vi "Database Query Search With Return Value.vi"(8 "error in (no error)":errorcluster, 10 "SQL query":string, 11 "object in":refnum<class "Database.lvclass">) -> (0 "error out":errorcluster, 1 "Not Empty":bool, 2 "recordset data":variant[][](array[variant]), 3 "object out":refnum<class "Database.lvclass">)   [LabVIEW 2015, in "Database.lvclass"]
uses:
  Database.lvclass
  <vilib>/addons/database/Auxilliary.llb/DB Tools Cursor Type.ctl
  Database.lvclass/Database.ctl
  <vilib>/addons/database/Connection.llb/DB Tools Open Connec (String).vi
  <vilib>/addons/database/Connection.llb/Conn Execute.vi
  <vilib>/addons/database/Recordset.llb/Rec Get Recordset Properties (R).vi
  <vilib>/addons/database/Recordset.llb/Rec Fetch Recordset Data (R).vi
  <vilib>/addons/database/Recordset.llb/Rec Destroy - Connection.vi
  <vilib>/addons/database/NI_Database_API.lvlib
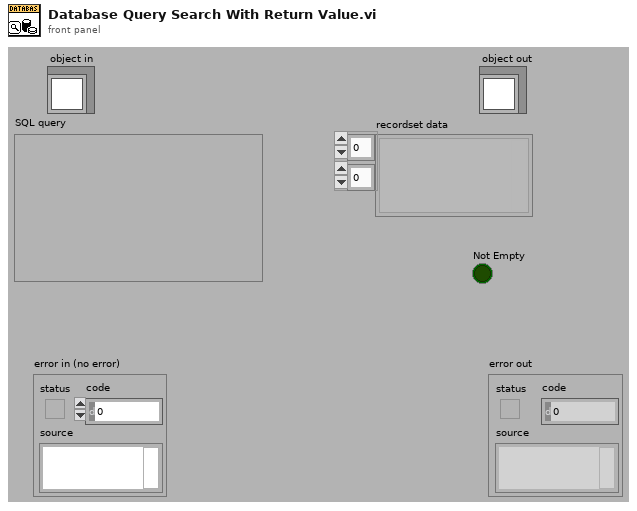
[diagram p1: front panel]
types:
  T1 = typedef "NI_Database_API.lvlib/DB Tools Cursor Type.ctl" = enum16{"forward-only", "keyset", "dynamic", "static"}
  T2 = typedef "NI_Database_API.lvlib/Conn ObjectReference.ctl" = refnum<k1>
  T3 = typedef "NI_Database_API.lvlib/Rec ObjectReference.ctl" = refnum<k1>
  T4 = typedef "NI_Database_API.lvlib/Rec Properties.ctl" = cluster{"column count":i32, "record index":i32, "record count":i32, "bof?":bool, "eof?":bool, "cursor type":T1, "cache size":i32, "state":enum16{"closed", "open"}}
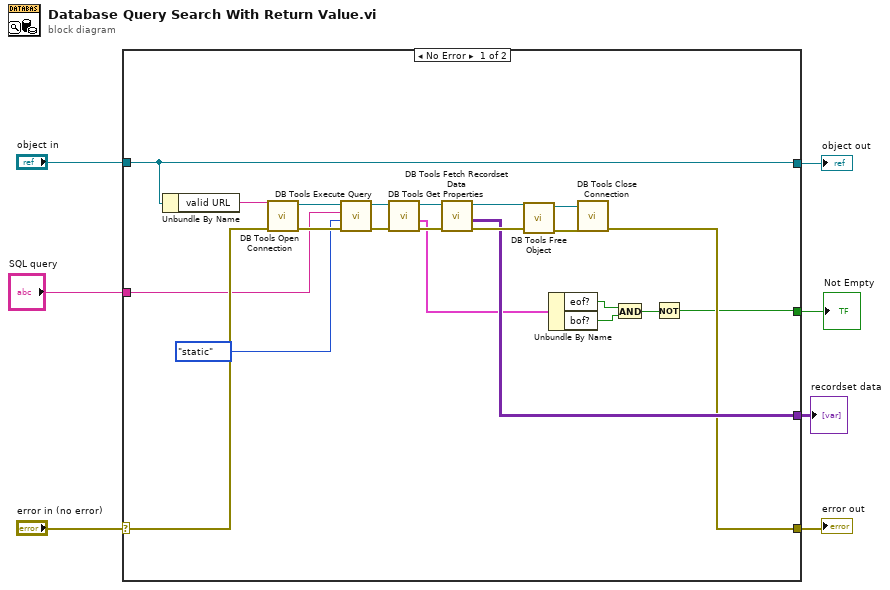
[diagram p0: block diagram]
diagram:
  n1 = case shown="No Error" "error in (no error)" {
    selector: "error in (no error)" -> [w27 w31]
    tunnel: [w17 w31] -> w6
    tunnel: [w29 w30] -> w4
    tunnel: "object in" -> [w29 w30]
    tunnel: "SQL query" -> [w23 _]
    tunnel: [w18 _] -> w2
    tunnel: [w8 _] -> w1
    frame No Error {
      n2 = Unbundle By Name(w29) -> ("valid URL"=w28:string)
      n3 = call-poly <vilib>:"DB Tools Open Connection.vi"("error in (no error)"=w27, "connection information"=w28) -> ("error out"=w25:errorcluster, "connection reference"=w26:T2)  [unwired: 6 in]
      n4 = call-poly <vilib>:"DB Tools Execute Query.vi"("error in (no error)"=w25, "cursor type"=DB_Tools_Cursor_Type."static", "SQL query"=w23, "connection reference"=w26) -> ("error out"=w15:errorcluster, "recordset reference"=w16:T3)  [unwired: 4 in]
      n5 = call-poly <vilib>:"DB Tools Get Properties.vi"("error in (no error)"=w15, "recordset reference"=w16) -> ("error out"=w13:errorcluster, "recordset properties"=w12:T4, "recordset reference out"=w14:T3)  [unwired: 3 in]
      n6 = call-poly <vilib>:"DB Tools Fetch Recordset Data.vi"("error in (no error)"=w13, "recordset reference"=w14) -> ("error out"=w19:errorcluster, "recordset data"=w18:variant[][], "recordset reference out"=w20:T3)  [unwired: 3 in]
      n7 = call-poly <vilib>:"DB Tools Free Object.vi"("error in (no error)"=w19, "recordset reference"=w20) -> ("error out"=w22:errorcluster, "connection reference"=w21:T2)  [unwired: 8 in]
      n8 = Unbundle By Name(w12) -> ("eof?"=w11:bool, "bof?"=w10:bool)
      n9 = call <vilib>:"DB Tools Close Connection.vi"("error in (no error)"=w22, "connection reference"=w21) -> ("error out"=w17:errorcluster)  [unwired: 5 in]
      n10 = And(x=w11, y=w10) -> (x .and. y?=w9:bool)
      n11 = Not(x=w9) -> (.not. x?=w8:bool)
    }
    frame Error {
    }
  }
  "error out" <- w6
  "object out" <- w4
  "recordset data" <- w2
  "Not Empty" <- w1
